vi "Vision Turning.vi"(0 "Speed 1":dbl=0.55, 1 "Range 1":dbl=0.75, 2 "Speed 2":dbl=0.45, 3 "Range 2":dbl=0.05) -> (6 "Motor Output":dbl, 7 "Boolean":bool, 8 "Vision In Range":bool, 9 "Scaled Vision X":dbl=0.11093750000000008, 10 "Final Range":dbl=0.05)   [LabVIEW 2015]
uses:
  <vilib>/Rock Robotics/WPI/Utilities/WPI_GetSetVariantRefNum.vi
  Code/Robot Global Data.vi
  <vilib>/Rock Robotics/WPI/RobotDrive/WPI_RobotDriveArcadeDrive_Standard(NoSaturation).vi
panel:
  in  "Vision Value":dbl
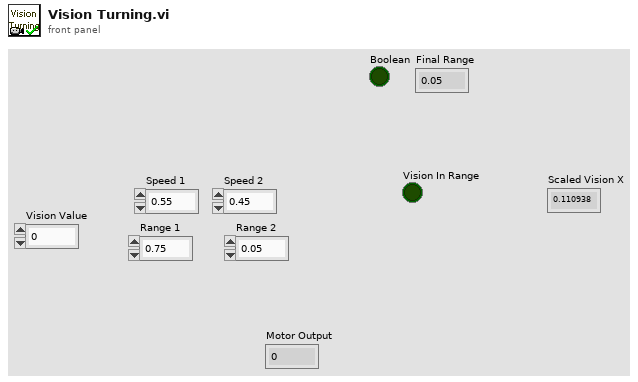
[diagram p1: front panel]
types:
  T1 = typedef "WPI_RobotDriveDevRef.ctl" = cluster{"DevStatus":errorcluster, "Motors[]":T2[], "Square Inputs":bool, "Max Output":dbl}
  T2 = typedef "WPI_MotorControlDeviceRef.ctl" = cluster{"DeviceStatus":errorcluster, "Type":T3, "PWM":cluster{"PWM Channel":T4, "DeadBand":T5}, "CAN":cluster{"Device Number":u8, "Control Mode":T6, "Semaphore":T7, "Max Vout":dbl, "TalonSRX Control Mode":T8}, "Invert":bool}
  T3 = typedef "WPI_MotorControlType.ctl" = enum16{"PWM", "CAN", "CANTalonSRX"}
  T4 = typedef "FPGA_DIOPWMChannel.ctl" = enum8{"PWM 0", "PWM 1", "PWM 2", "PWM 3", "PWM 4", "PWM 5", "PWM 6", "PWM 7", "PWM 8", "PWM 9", "PWM MXP 0", "PWM MXP 1", "PWM MXP 2", "PWM MXP 3", "PWM MXP 4", "PWM MXP 5", "PWM MXP 6", "PWM MXP 7", "PWM MXP 8", "PWM MXP 9", "Invalid"}
  T5 = typedef "WPI_PWMDeadband.ctl" = cluster{"Name":string, "maxPositivePwm":i32, "minPositivePwm":i32, "centerPwm":i32, "maxNegativePwm":i32, "minNegativePwm":i32, "angularRange":u16}
  T6 = typedef "WPI_CANJaguar_ControlMode.ctl" = enum8{"Percent VBus", "Current", "Speed", "Position", "Voltage"}
  T7 = typedef "Semaphore RefNum" = refnum<k1>
  T8 = typedef "WPI_CANTalonSRX_APIControlMode.ctl" = enum8{"Percent VBus", "Speed", "Position", "Slave", "Unchanged / Invalid", "Voltage Compensation", "Current", "Motion Profile"}
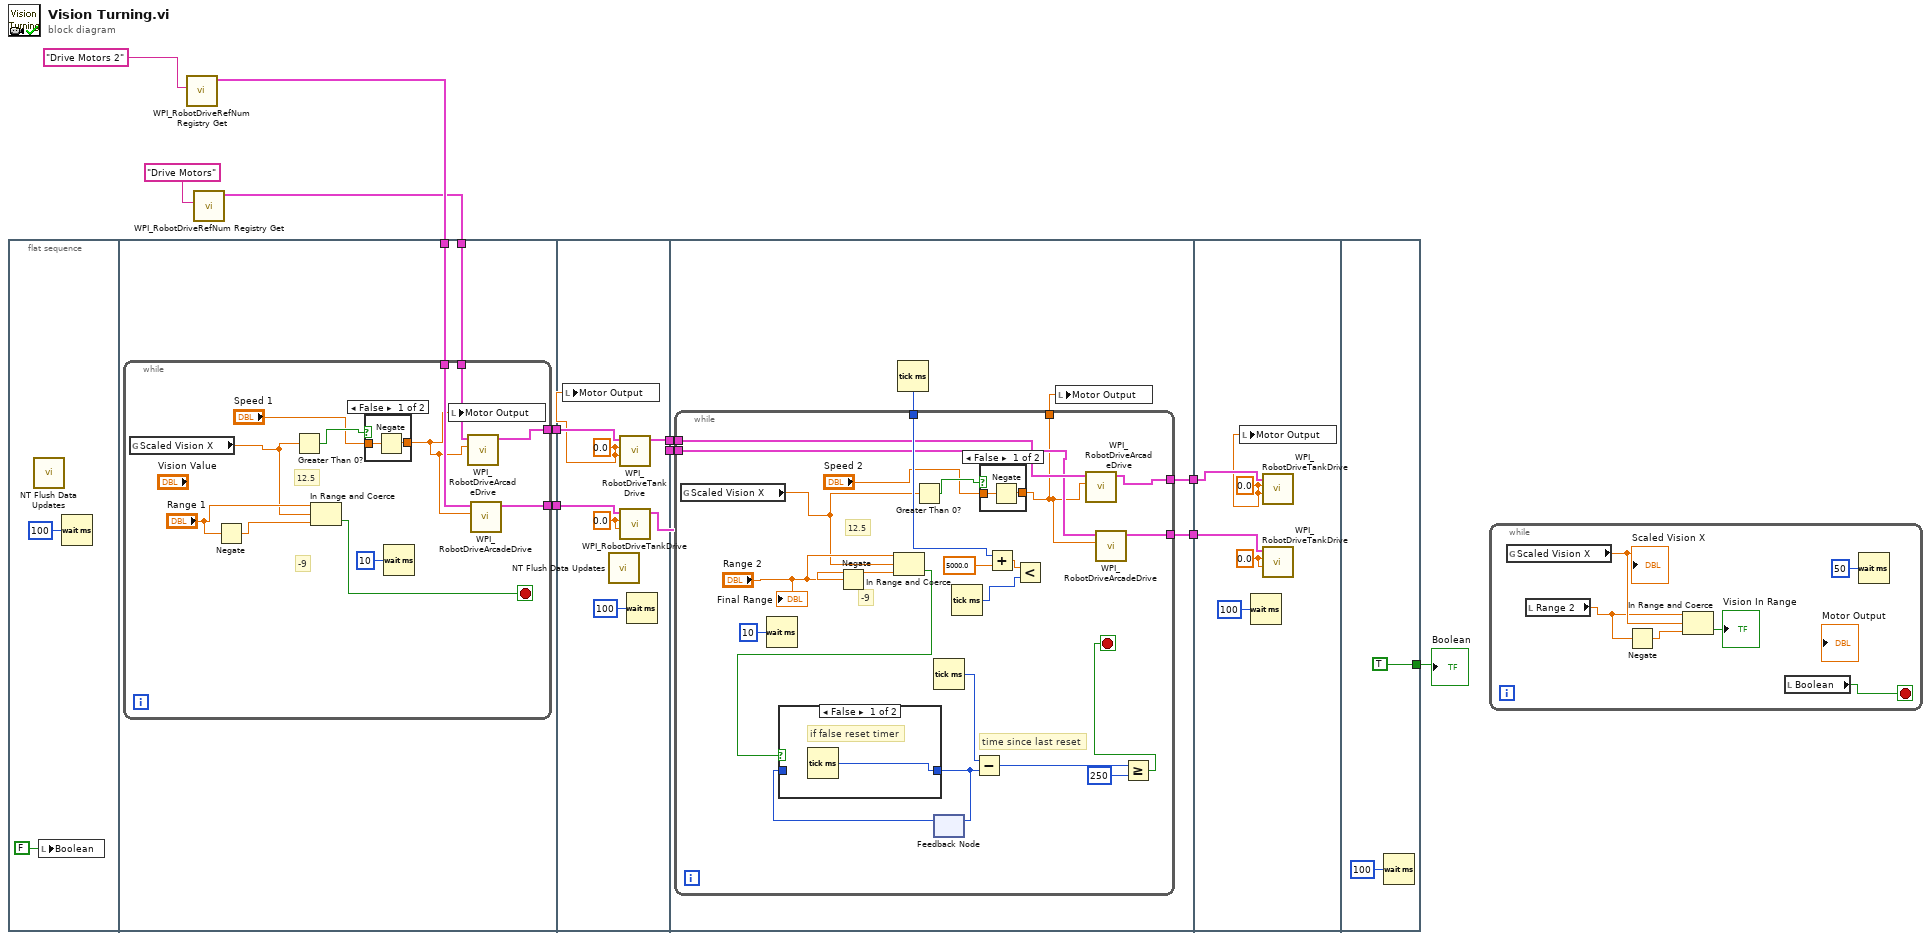
[diagram p0: block diagram]
diagram:
  n1 = flat-sequence {
    tunnel: [w17] -> w11
    tunnel: w5 -> [w16]
    tunnel: w6 -> [w15]
    tunnel: [w14] -> w4
    tunnel: [w38] -> w10
    tunnel: [w37] -> w3
    tunnel: w4 -> [w34]
    tunnel: w11 -> [w36]
    tunnel: w10 -> [w45]
    tunnel: [w44] -> w9
    tunnel: w3 -> [w42]
    tunnel: [w41] -> w2
    tunnel: w2 -> [w74]
    tunnel: w9 -> [w75]
    tunnel: [TRUE] -> w1
    frame #0 {
      n2 = call <vilib>:"NT Flush Data Updates.vi"() -> ()  [unwired: 11 in, 1 out]
      n3 = local write "Boolean"(FALSE ("Boolean")) -> ()
      n4 = Wait (ms)(milliseconds to wait=u32 100) -> ()  [unwired: 1 out]
    }
    frame #1 {
      n5 = while {
        tunnel: [w26] -> w17
        tunnel: w16 -> [w25]
        tunnel: w15 -> [w24]
        tunnel: [w23] -> w14
        stop <- w27 stop-if-true
        # "-9"
        # "12.5"
        n6 = global read "Robot Global Data.vi" "Scaled Vision X"() -> (w19:dbl)
        n7 = Negate(x="Range 1") -> (-x=w21:dbl)
        n8 = Greater Than 0?(x=w19) -> (x > 0?=w28:bool)
        n9 = In Range and Coerce(upper limit="Range 1", x=w19, lower limit=w21) -> (In Range?=w27:bool)  [unwired: 1 out]
        n10 = case shown="False" w28 {
          tunnel: "Speed 1" -> [w31 w32]
          tunnel: [w30 w32] -> w18
          frame False {
            n11 = Negate(x=w31) -> (-x=w30:dbl)
          }
          frame True {
          }
        }
        n12 = Wait (ms)(milliseconds to wait=u32 10) -> ()  [unwired: 1 out]
        n13 = local write "Motor Output"(w18) -> ()
        n14 = call-poly <vilib>:"WPI_RobotDriveArcadeDrive.vi"("X axis value"=w18, "RobotDriveDevRef"=w25) -> ("RobotDriveDevRef"=w26:T1)  [unwired: 7 in, 2 out]
        n15 = call-poly <vilib>:"WPI_RobotDriveArcadeDrive.vi"("X axis value"=w18, "RobotDriveDevRef"=w24) -> ("RobotDriveDevRef"=w23:T1)  [unwired: 7 in, 2 out]
      }
    }
    frame #2 {
      w35 = 0.0 ("Left axis value")
      w33 = 0.0 ("Left axis value")
      n16 = local write "Motor Output"(w33) -> ()
      n17 = call <vilib>:"NT Flush Data Updates.vi"() -> ()  [unwired: 11 in, 1 out]
      n18 = call <vilib>:"WPI_RobotDriveTankDrive.vi"("Right axis value"=w33, "Left axis value"=w33, "RobotDriveDevRef"=w36) -> ("RobotDriveDevRef"=w38:T1)  [unwired: 6 in, 2 out]
      n19 = call <vilib>:"WPI_RobotDriveTankDrive.vi"("Right axis value"=w35, "Left axis value"=w35, "RobotDriveDevRef"=w34) -> ("RobotDriveDevRef"=w37:T1)  [unwired: 6 in, 2 out]
      n20 = Wait (ms)(milliseconds to wait=u32 100) -> ()  [unwired: 1 out]
    }
    frame #3 {
      n21 = Tick Count (ms)() -> (millisecond timer value=w43:u32)
      n22 = while {
        tunnel: w45 -> [w60]
        tunnel: [w61] -> w44
        tunnel: w43 -> [w64]
        tunnel: w42 -> [w59]
        tunnel: [w58] -> w41
        tunnel: [w53] -> w40
        stop <- w47 stop-if-true
        # "time since last reset"
        # "-9"
        # "12.5"
        n23 = global read "Robot Global Data.vi" "Scaled Vision X"() -> (w54:dbl)
        n24 = Wait (ms)(milliseconds to wait=u32 10) -> ()  [unwired: 1 out]
        n25 = Negate(x="Range 2") -> (-x=w57:dbl)
        n26 = In Range and Coerce(upper limit="Range 2", x=w54, lower limit=w57) -> (In Range?=w48:bool)  [unwired: 1 out]
        n27 = Greater Than 0?(x=w54) -> (x > 0?=w66:bool)
        n28 = Tick Count (ms)() -> (millisecond timer value=w52:u32)
        n29 = feedback #1() -> (w51:u32)  [unwired: 1 in]
        n30 = case shown="False" w48 {
          tunnel: [w68 w69] -> w50
          tunnel: w51 -> [_ w69]
          frame False {
            # "if false reset timer"
            n31 = Tick Count (ms)() -> (millisecond timer value=w68:u32)
          }
          frame True {
            # "if true don't reset timer"
          }
        }
        n32 = feedback-in #1(w50) -> ()
        n33 = Tick Count (ms)() -> (millisecond timer value=w63:u32)
        n34 = Subtract(x=w52, y=w50) -> (x-y=w49:u32)
        n35 = case shown="False" w66 {
          tunnel: "Speed 2" -> [w71 w72]
          tunnel: [w70 w72] -> w53
          frame False {
            n36 = Negate(x=w71) -> (-x=w70:dbl)
          }
          frame True {
          }
        }
        n37 = Add(x=w64, y=5000.0) -> (x+y=w62:dbl)
        n38 = Less?(x=w62, y=w63) -> ()  [unwired: 1 out]
        n39 = call-poly <vilib>:"WPI_RobotDriveArcadeDrive.vi"("X axis value"=w53, "RobotDriveDevRef"=w60) -> ("RobotDriveDevRef"=w61:T1)  [unwired: 7 in, 2 out]
        n40 = call-poly <vilib>:"WPI_RobotDriveArcadeDrive.vi"("X axis value"=w53, "RobotDriveDevRef"=w59) -> ("RobotDriveDevRef"=w58:T1)  [unwired: 7 in, 2 out]
        n41 = Greater Or Equal?(x=w49, y=u32 250) -> (x >= y?=w47:bool)
        "Final Range" <- "Range 2"
      }
      n42 = local write "Motor Output"(w40) -> ()
    }
    frame #4 {
      w76 = 0.0 ("Left axis value")
      w73 = 0.0 ("Left axis value")
      n43 = local write "Motor Output"(w73) -> ()
      n44 = Wait (ms)(milliseconds to wait=u32 100) -> ()  [unwired: 1 out]
      n45 = call <vilib>:"WPI_RobotDriveTankDrive.vi"("Right axis value"=w73, "Left axis value"=w73, "RobotDriveDevRef"=w75) -> ()  [unwired: 6 in, 3 out]
      n46 = call <vilib>:"WPI_RobotDriveTankDrive.vi"("Right axis value"=w76, "Left axis value"=w76, "RobotDriveDevRef"=w74) -> ()  [unwired: 6 in, 3 out]
    }
    frame #5 {
      n47 = Wait (ms)(milliseconds to wait=u32 100) -> ()  [unwired: 1 out]
    }
  }
  n48 = call <vilib>:"WPI_RobotDriveRefNum Registry Get.vi"("refnum name"="Drive Motors 2") -> ("RobotDriveDevRef"=w6:T1)  [unwired: 1 in, 9 out]
  n49 = call <vilib>:"WPI_RobotDriveRefNum Registry Get.vi"("refnum name"="Drive Motors") -> ("RobotDriveDevRef"=w5:T1)  [unwired: 1 in, 9 out]
  n50 = while {
    stop <- w85 stop-if-true
    n51 = global read "Robot Global Data.vi" "Scaled Vision X"() -> (w83:dbl)
    "Scaled Vision X" <- w83
    n52 = local read "Range 2"() -> (w81:dbl)
    n53 = Negate(x=w81) -> (-x=w82:dbl)
    n54 = In Range and Coerce(upper limit=w81, x=w83, lower limit=w82) -> (In Range?=→"Vision In Range":bool)  [unwired: 1 out]
    n55 = local read "Boolean"() -> (w85:bool)
    n56 = Wait (ms)(milliseconds to wait=u32 50) -> ()  [unwired: 1 out]
  }
  "Boolean" <- w1
